vi "WaitOnProcessSync.vi"(7 "Wait for start? (T)":bool=TRUE, 8 "error in (no error)":errorcluster, 9 "timeout in ms (-1)":i32=-1, 11 "SMO":refnum<class "SMO.lvclass">) -> (0 "error out":errorcluster, 1 "Don't run?":bool, 3 "SMO out":refnum<class "SMO.lvclass">)   [LabVIEW 2013, in "SMO.lvclass"]
doc: "This method is used to synchronize processes during launch and shutdown\n\nNote: This method is overridable by descendant\n\n---------------------------------------------------------------\nJKI State Machine Objects™\nhttp://jki.net/state-machine-objects/\nCopyright (C) 2005-2015, JKI <info@jki.net>\nALL RIGHTS RESERVED"
uses:
  SMO.lvclass
  Typedefs/SMOState --Enum.ctl
  SMO.lvclass/SMO.ctl
  Private/ReftoDVR--SMO.vi
  Private/DVRtoRef--SMO.vi
  <vilib>/Utility/error.llb/Error Cluster From Error Code.vi
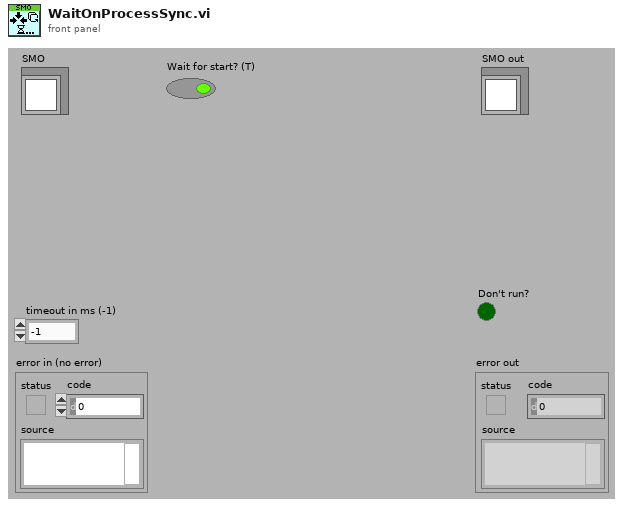
[diagram p1: front panel]
types:
  T1 = typedef "SMO.lvclass/SMOState --Enum.ctl" = enum16{"unknown", "Created", "Started", "Stopped"}
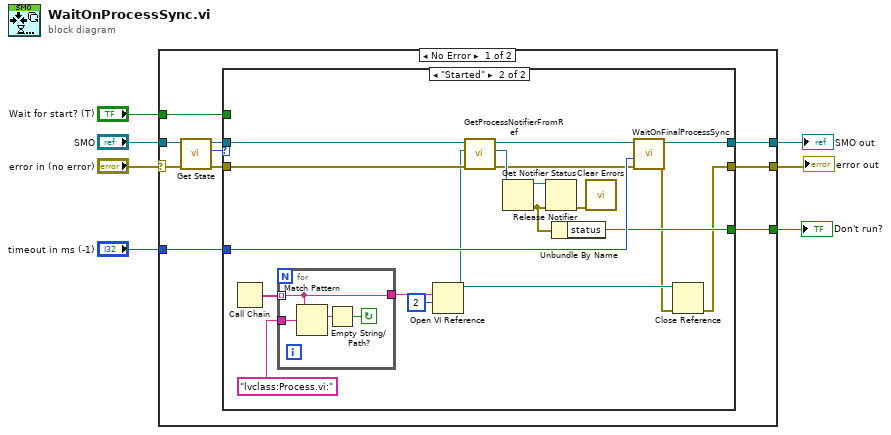
[diagram p0: block diagram]
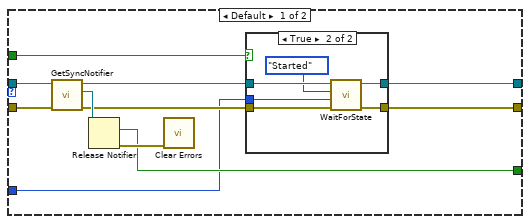
[diagram p2: hidden frame]
diagram:
  n1 = case shown="No Error" "error in (no error)" {
    selector: "error in (no error)" -> [w16 w60]
    tunnel: [w14 w60] -> w6
    tunnel: [w15 w59] -> w5
    tunnel: "SMO" -> [w17 w59]
    tunnel: "timeout in ms (-1)" -> [w13 _]
    tunnel: [w9 _] -> w2
    tunnel: "Wait for start? (T)" -> [w8 _]
    frame No Error {
      n2 = call "Get State.vi"("error in (no error)"=w16, "SMO"=w17) -> ("error out"=w11:errorcluster, "SMO State"=w10:T1, "SMO out"=w12:refnum<class "SMO.lvclass">)  [unwired: 7 in]
      n3 = case shown="\"Started\"" w10 {
        tunnel: [w22 w53] -> w15
        tunnel: [w20 w40] -> w14
        tunnel: w12 -> [w26 w49]
        tunnel: w11 -> [w27 w47]
        tunnel: w13 -> [w19 w54]
        tunnel: [w24 w44] -> w9
        tunnel: w8 -> [w18 _]
        frame Default {
          n4 = call "GetSyncNotifier.vi"("error in (no error)"=w27, "SMO in"=w26) -> ("error out"=w21:errorcluster, "Sync Notifier"=w28:refnum<notifier>, "SMO out"=w23:refnum<class "SMO.lvclass">)  [unwired: 7 in]
          n5 = Release Notifier(notifier=w28) -> (last notification=w24:bool, error out=w25:errorcluster)  [unwired: 2 in, 1 out]
          n6 = call <vilib>:"Clear Errors.vi"("error in (no error)"=w25) -> ()  [unwired: 6 in, 1 out]
          n7 = case shown="True" w18 {
            tunnel: w23 -> [w30 w36]
            tunnel: [w30 w35] -> w22
            tunnel: w21 -> [w29 w34]
            tunnel: [w29 w33] -> w20
            tunnel: w19 -> [_ w32]
            frame False {
            }
            frame True {
              n8 = call "WaitForState.vi"("error in (no error)"=w34, "timeout in ms (-1)"=w32, "State (unknown: any state)"=SMOState_--Enum."Started", "SMO in"=w36) -> ("error out"=w33:errorcluster, "SMO out"=w35:refnum<class "SMO.lvclass">)  [unwired: 5 in, 1 out]
            }
          }
        }
        frame "Started" {
          n9 = Call Chain() -> (call chain=w39:string[])
          n10 = for {
            tunnel: w39 -> [w55] mode=indexing
            tunnel: "lvclass:Process.vi:" -> [w58]
            tunnel: [w55] -> w38
            stop <- w56 continue-if-true
            n11 = Match Pattern(string=w55, regular expression=w58) -> (match substring=w57:string)  [unwired: 1 in, 3 out]
            n12 = Empty String/Path?(string/path=w57) -> (empty?=w56:bool)
          }
          n13 = Open VI Reference(vi path=w38, options=2) -> (vi reference=w42:refnum<vi>)  [unwired: 4 in, 1 out]
          n14 = call "GetProcessNotifierFromRef.vi"("error in (no error)"=w47, "Process VI Refnum"=w42, "SMO"=w49) -> ("error out"=w46:errorcluster, "Sync Notifier"=w50:refnum<notifier>, "SMO out"=w48:refnum<class "SMO.lvclass">)  [unwired: 6 in]
          n15 = Get Notifier Status(notifier=w50) -> (notifier out=w52:refnum<notifier>, error out=w45:errorcluster)  [unwired: 1 in, 3 out]
          n16 = Release Notifier(notifier=w52, error in (no error)=w45) -> (error out=w43:errorcluster)  [unwired: 1 in, 2 out]
          n17 = Unbundle By Name(w45) -> ("status"=w44:bool)
          n18 = call <vilib>:"Clear Errors.vi"("error in (no error)"=w43) -> ()  [unwired: 6 in, 1 out]
          n19 = call "WaitOnFinalProcessSync.vi"("error in (no error)"=w46, "timeout in ms (-1)"=w54, "SMO"=w48) -> ("error out"=w41:errorcluster, "SMO out"=w53:refnum<class "SMO.lvclass">)  [unwired: 7 in]
          n20 = Close Reference(reference=w42, error in (no error)=w41) -> (error out=w40:errorcluster)
        }
      }
    }
    frame Error {
    }
  }
  "error out" <- w6
  "SMO out" <- w5
  "Don't run?" <- w2
